vi "Find in Constants Map.vi"(10 "Constant Name":string, 11 "Constants Map":T1) -> (0 "index":i32, 1 "Hash Index":i32, 2 "Did it find it":bool, 3 "Constants":T2)   [LabVIEW 2013]
uses:
  Constants typedef V2.ctl
  Constants Map typedef.ctl
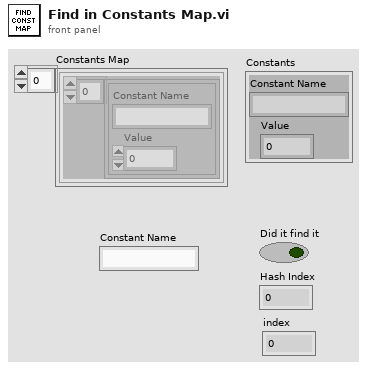
[diagram p1: front panel]
types:
  T1 = typedef "Constants Map typedef.ctl" = cluster{T2[]}[]
  T2 = typedef "Constants typedef V2.ctl" = cluster{"Constant Name":string, "Value":dbl}
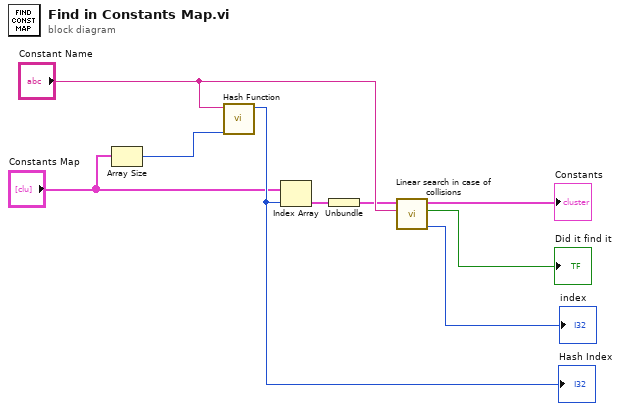
[diagram p0: block diagram]
diagram:
  n1 = Array Size(array="Constants Map") -> (size(s)=w3:i32)
  n2 = call "Hash Function.vi"("num Buckets"=w3, "Constant Name"="Constant Name") -> ("Hash Code"=w5:i32)  [unwired: 9 in]
  "Hash Index" <- w5
  n3 = Index Array(array="Constants Map", index=w5) -> (element=w2:cluster{T2[]})
  n4 = Unbundle(w2) -> (w1:T2[])
  n5 = call "Linear search in case of collisions.vi"("Constant Name"="Constant Name", "Array"=w1) -> ("index"=→"index":i32, "Did it find it"=→"Did it find it":bool, "Constants"=→"Constants":T2)  [unwired: 7 in]
